vi "start.vi"() -> ()   [LabVIEW 2014]
panel:
  out "布尔":bool
  out "Current Status":string
  out "Loading App":u8(slide) scale=0.0..26.0
  out "通知":string
  # "Version: C.1.0\n--\n南京天创智能     所有, 2017"
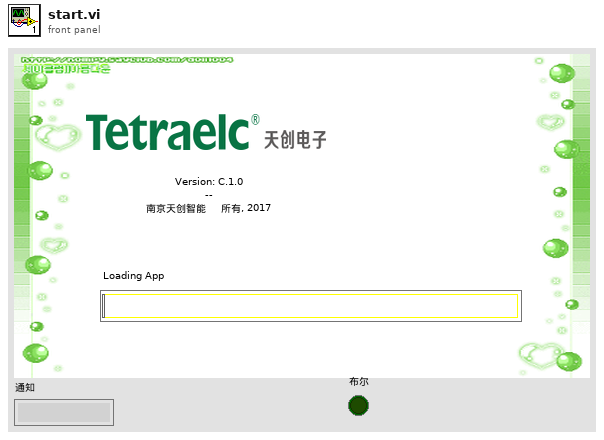
[diagram p1: front panel]
types:
  T1 = enum32{"Invalid", "Standard", "Closed", "Hidden", "Minimized", "Maximized"}
  T2 = enum32{"invalid app kind", "Development System", "Run Time System", "Student Edition", "Embedded LabVIEW", "Evaluation", "Custom"}
  T3 = enum32{"Bad", "Idle", "Run top level", "Running"}
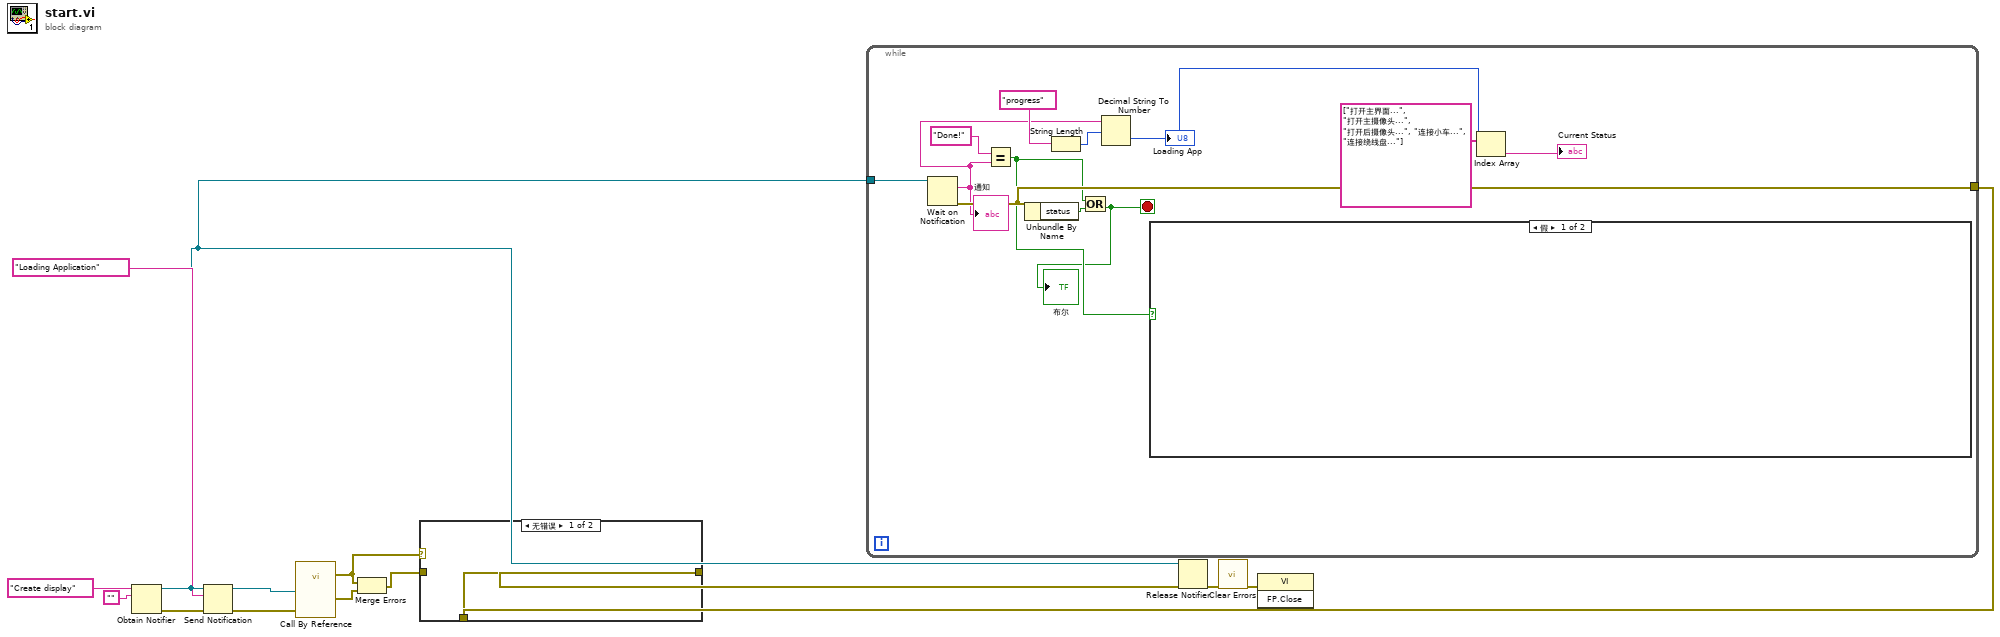
[diagram p0: block diagram]
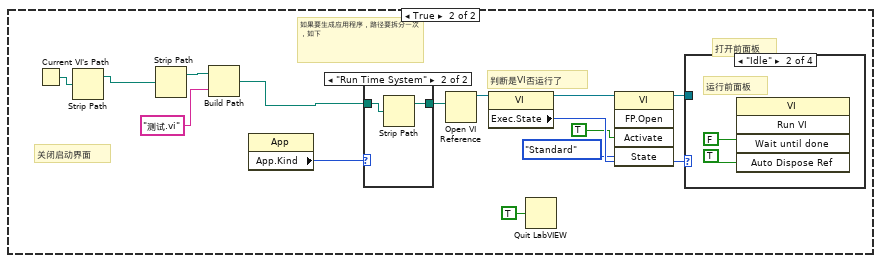
[diagram p2: hidden frame]
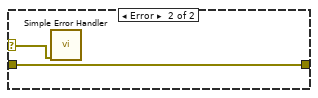
[diagram p7: hidden frame]
diagram:
  n1 = Obtain Notifier(name (unnamed)="Create display" ("名称（未命名）"), notification data type="") -> (notifier out=w4:refnum<notifier>, error out=w10:errorcluster)  [unwired: 2 in, 1 out]
  n2 = Send Notification(notification="Loading Application", notifier=w4, error in (no error)=w10) -> (notifier out=w1:refnum<notifier>, error out=w6:errorcluster)
  n3 = call-by-ref "?"(error in=w6, 1:"error in (no error)"=w6, "状态通知器"=w1) -> (error out=w7:errorcluster, 0:"error out"=w2:cluster{"状态":bool, "代码":i32, "源":string})  [unwired: 1 in, 1 out]
  n4 = Merge Errors(w7, w2) -> (w8:errorcluster)
  n5 = while {
    tunnel: w4 -> [w24]
    tunnel: [w23] -> w3
    stop <- w15 stop-if-true
    n6 = Wait on Notification(notifier=w24) -> (notification=w21:string, error out=w23:errorcluster)  [unwired: 3 in, 2 out]
    "通知" <- w21
    n7 = Equal?(x="Done!" ("notification"), y=w21) -> (x = y?=w16:bool)
    n8 = Unbundle By Name(w23) -> ("status"=w25:bool)
    n9 = String Length(string="progress" ("搜索字符串/字符(-)")) -> (length=w20:i32)
    n10 = Or(x=w16, y=w25) -> (x .or. y?=w15:bool)
    "布尔" <- w15
    n11 = Decimal String To Number(string=w21, offset=w20) -> (number=w17:i32)  [unwired: 1 in, 1 out]
    "Loading App" <- w17
    n12 = case shown="假" w16 {
      frame False {
      }
      frame True {
        # "如果要生成应用程序，路径要拆分一次，如下"
        # "判断是VI否运行了"
        # "打开前面板"
        # "关闭启动界面"
        n13 = Current VI's Path() -> (path=w38:path)
        n14 = Strip Path(path=w38) -> (stripped path=w37:path)  [unwired: 1 out]
        n15 = Strip Path(path=w37) -> (stripped path=w40:path)  [unwired: 1 out]
        n16 = Build Path(base path=w40, name or relative path="测试.vi" ("名称或相对路径")) -> (appended path=w28:path)
        n17 = property class="App"() -> ("App.Kind"=w30:T2)  [unwired: 2 in, 2 out]
        n18 = case shown="\"Run Time System\"" w30 {
          tunnel: [w41 w42] -> w29
          tunnel: w28 -> [w41 w43]
          frame "Development System", Default {
          }
          frame "Run Time System" {
            n19 = Strip Path(path=w43) -> (stripped path=w42:path)  [unwired: 1 out]
          }
        }
        n20 = Open VI Reference(vi path=w29) -> (vi reference=w36:refnum<vi>)  [unwired: 5 in, 1 out]
        n21 = property class="VI"(reference=w36) -> (reference out=w32:refnum<vi>, "Exec.State"=w35:T3)  [unwired: 1 in, 1 out]
        n22 = Quit LabVIEW(quit? (T)=TRUE ("退出？(T)")) -> ()
        n23 = invoke class="VI" method="FP.Open"(reference=w32, "Activate"=TRUE ("Activate?"), "State"=T1."Standard") -> (reference out=w31:refnum<vi>)  [unwired: 2 in, 4 out]
        n24 = case shown="\"Idle\"" w35 {
          tunnel: w31 -> [_ _ _ _]
          frame "Bad", Default {
          }
          frame "Idle" {
            # "运行前面板"
            n25 = invoke class="VI" method="Run VI"("Wait until done"=FALSE ("结束前等待"), "Auto Dispose Ref"=TRUE ("自动销毁引用")) -> ()  [unwired: 3 in, 5 out]
          }
          frame "Run top level" {
          }
          frame "Running" {
          }
        }
      }
    }
    n26 = Index Array(array=string[] ["打开主界面...", "打开主摄像头...", "打开后摄像头...", "连接小车...", "连接绕线盘..."], index=w17) -> (element=→"Current Status":string)
  }
  n27 = case shown="无错误" w7 {
    tunnel: [w46 w47] -> w9
    tunnel: w8 -> [_ w47]
    selector: w7 -> [_ w48]
    tunnel: w3 -> [w46 _]
    frame No Error {
    }
    frame Error {
      n28 = call <vilib>:"Simple Error Handler.vi"("error in (no error)"=w48) -> ()  [unwired: 4 in, 5 out]
    }
  }
  n29 = Release Notifier(notifier=w4, error in (no error)=w9) -> (error out=w14:errorcluster)  [unwired: 1 in, 2 out]
  n30 = call <vilib>:"Clear Errors.vi"("error in (no error)"=w14) -> ("error out"=w11:errorcluster)  [unwired: 5 in, 1 out]
  n31 = invoke class="VI" method="FP.Close"(error in=w11) -> ()  [unwired: 2 in, 3 out]
